vi "MotorControlExample.vi"() -> ()   [LabVIEW 2019, in "CubeMarsBLDClib.lvlib"]
uses:
  CubeMarsBLDClib.lvlib
  MotorParameters.ctl
  Reference.ctl
  MotorType.ctl
  ReadMotorData.ctl
  <vilib>/myRIO/Common/Instrument Driver Framework/myRIO v1.0/UART/vis/myRIO v1.0 Close UART.vi
  <vilib>/myRIO/Common/Instrument Driver Framework/Utilities/vis/FPGA Ref Manager.vi
  <vilib>/myRIO/Common/Instrument Driver Framework/myRIO v1.0/myRIO v1.0 Reset FPGA.vi
  <vilib>/myRIO/Common/Instrument Driver Framework/myRIO v1.0/IRQ/vis/myRIO v1.0 IRQ Info FGV.vi
  <vilib>/myRIO/Common/Instrument Driver Framework/myRIO v1.0/IRQ/vis/myRIO v1.0 Timer IRQ Info FGV.vi
  <vilib>/myRIO/Common/Instrument Driver Framework/myRIO v1.0/IRQ/vis/myRIO v1.0 ISR Agent.vi
  <vilib>/myRIO/Instrument Drivers/Utilities/vis/Reset Index.vi
  <vilib>/myRIO/Common/Instrument Driver Framework/myRIO v1.0/Resource Manager/vis/myRIO v1.0 Block Write Resource Manager.vi
  <vilib>/myRIO/Instrument Drivers/Utilities/Utilities.lvlib
panel:
  out "ReadData":T4(array[cluster])
  in  "CAN ID":u32=1
  in  "Send CMD":bool=TRUE
  out "FilteredValue":T5
  out "dt(ms)":dbl
  in  "Disable Motor":bool
  in  "ValueIn":T5
  in  "Enable Motor":bool
  out "error out":errorcluster
  in  "stop":bool
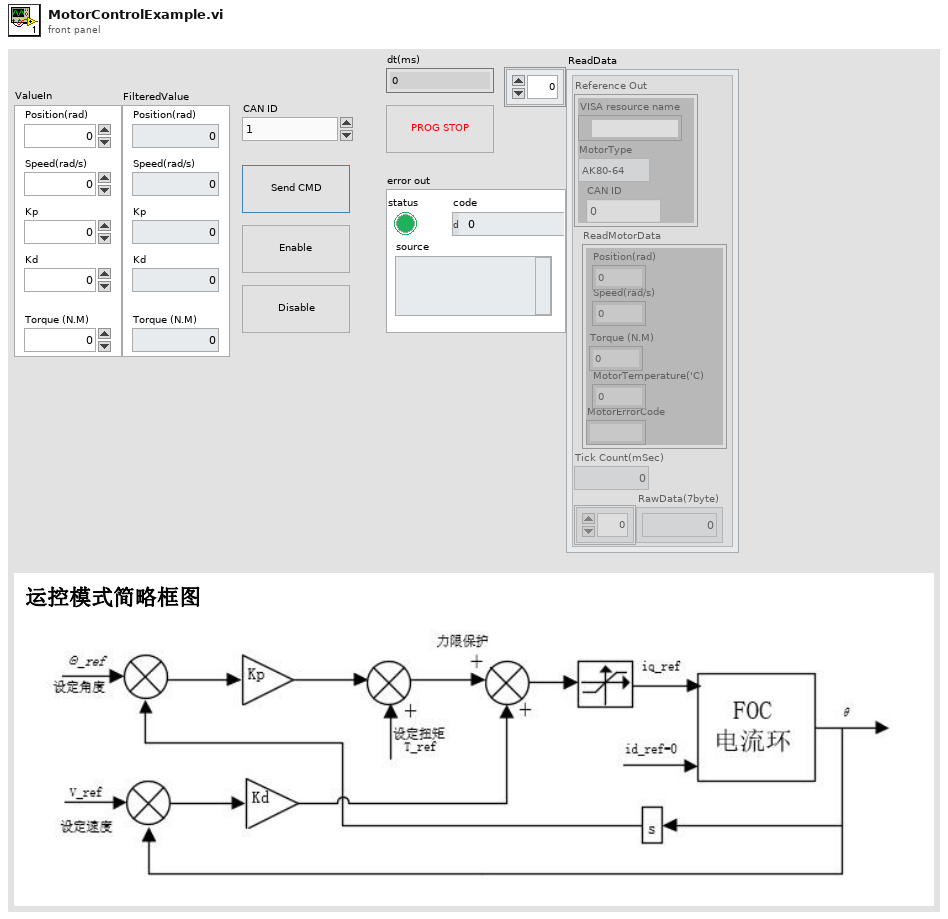
[diagram p1: front panel]
types:
  T1 = typedef "CubeMarsBLDClib.lvlib/Reference.ctl" = cluster{"VISA resource name":refnum<visa-resource-name>, "MotorType":T2, "CAN ID":u32}
  T2 = typedef "CubeMarsBLDClib.lvlib/MotorType.ctl" = enum16{"AK80-64", "AK80-9", "AK80-8", "AK80-6", "AK70-10", "AK60-6", "AK10-9"}
  T3 = typedef "CubeMarsBLDClib.lvlib/ReadMotorData.ctl" = cluster{"Position(rad)":dbl, "Speed(rad/s)":dbl, "Torque (N.M)":dbl, "MotorTemperature('C)":sgl, "MotorErrorCode":string}
  T4 = cluster{"Reference Out":T1, "ReadMotorData":T3, "Tick Count(mSec)":u32, "RawData(7byte)":u8[]}[]
  T5 = typedef "CubeMarsBLDClib.lvlib/MotorParameters.ctl" = cluster{"Position(rad)":dbl, "Speed(rad/s)":dbl, "Kp":dbl, "Kd":dbl, "Torque (N.M)":dbl}
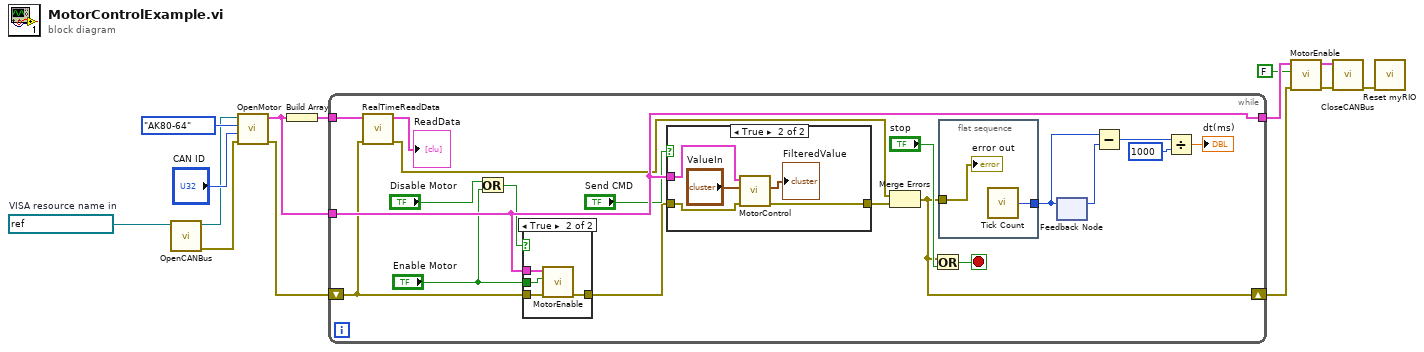
[diagram p0: block diagram]
diagram:
  w7 = refnum<visa-resource-name> "ASRL3::INSTR"  # VISA resource name in
  n1 = call "OpenCANBus.vi"("USB-CAN COM Port"=w7) -> ("Error Out"=w6:errorcluster, "VISA resource name out"=w8:refnum<visa-resource-name>)  [unwired: 9 in]
  n2 = call "OpenMotor.vi"("Error In"=w6, "CAN ID"="CAN ID", "MotorType"=MotorType."AK80-64", "USB CAN VISA resource name"=w8) -> ("Error Out"=w14:errorcluster, "Reference Out"=w12:T1)  [unwired: 6 in]
  n3 = Build Array(w12) -> (w11:T1[])
  n4 = while {
    shift-right: [w16] -> w5
    shift-left: w14 -> [w24]
    tunnel: w12 -> [w31]
    tunnel: [w31] -> w3
    tunnel: w11 -> [w25]
    stop <- w32 stop-if-true
    n5 = call "RealTimeReadData.vi"("error in"=w24, "AllMotorReference(Same port)"=w25) -> ("error out"=w23:errorcluster, "ReadData"=→"ReadData":T4)  [unwired: 8 in]
    n6 = Or(x="Disable Motor", y="Enable Motor") -> (x .or. y?=w20:bool)
    n7 = case shown="True" w20 {
      tunnel: w24 -> [w42 w46]
      tunnel: [w42 w45] -> w18
      tunnel: w31 -> [_ w44]
      tunnel: "Enable Motor" -> [_ w43]
      frame False {
      }
      frame True {
        n8 = call "MotorEnable.vi"("Error In"=w46, "Enable?(F)"=w43, "Reference In"=w44) -> ("Error Out"=w45:errorcluster)  [unwired: 7 in, 1 out]
      }
    }
    n9 = case shown="True" "Send CMD" {
      tunnel: [w36 w41] -> w22
      tunnel: w18 -> [w36 w40]
      tunnel: w31 -> [_ w39]
      frame False {
      }
      frame True {
        n10 = call "MotorControl.vi"("error in"=w40, "ValueIn"="ValueIn", "Reference In"=w39) -> ("error out"=w41:errorcluster, "FilteredValue"=→"FilteredValue":T5)  [unwired: 6 in, 1 out]
      }
    }
    n11 = Merge Errors(w23, w22) -> (w16:errorcluster)
    n12 = Or(x=w16, y="stop") -> (x .or. y?=w32:bool)
    n13 = flat-sequence {
      tunnel: [w35] -> w29
      tunnel: w16 -> [w34]
      frame #0 {
        n14 = call "Tick Count"() -> ("Tick Count(uSec)"=w35:u32)
        "error out" <- w34
      }
    }
    n15 = feedback #1() -> (w28:u32)  [unwired: 1 in]
    n16 = feedback-in #1(w29) -> ()
    n17 = Subtract(x=w29, y=w28) -> (x-y=w27:u32)
    n18 = Divide(x=w27, y=u32 1000) -> (x/y=→"dt(ms)":dbl)
  }
  n19 = call "MotorEnable.vi"("Error In"=w5, "Enable?(F)"=FALSE, "Reference In"=w3) -> ("Error Out"=w4:errorcluster, "Reference Out"=w2:T1)  [unwired: 7 in]
  n20 = call "CloseCANBus.vi"("Error In"=w4, "Reference In"=w2) -> ("Error Out"=w13:errorcluster)  [unwired: 9 in]
  n21 = call <vilib>:"Reset myRIO.vi"("error in (no error)"=w13) -> ()  [unwired: 10 in, 1 out]
